vi "Define Cells names.vi"(8 "error in (no error)":errorcluster, 11 "Control-Client in":refnum<class "Control-Client.lvclass">) -> (0 "error out":errorcluster, 3 "Control-Client out":refnum<class "Control-Client.lvclass">)   [LabVIEW 2019, in "Control-Client.lvclass"]
uses:
  Control-Client.lvclass
  Control-Client.lvclass/Control-Client.ctl
panel:
  in  "Names of cells":string[](array[string])
  in  "stop":bool
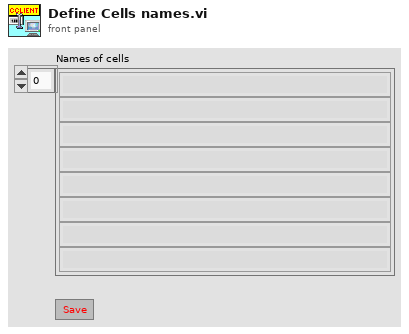
[diagram p1: front panel]
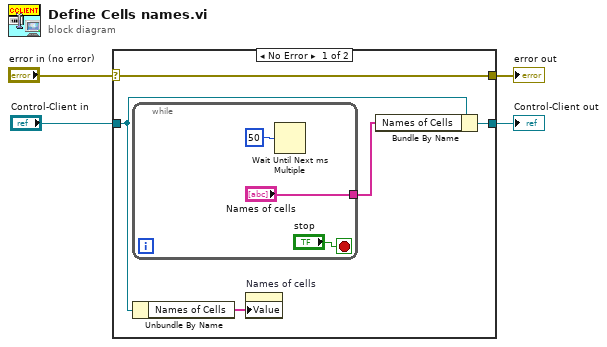
[diagram p0: block diagram]
diagram:
  n1 = case shown="No Error" "error in (no error)" {
    selector: "error in (no error)" -> [w9 w14]
    tunnel: [w9 w14] -> w3
    tunnel: [w5 w13] -> w1
    tunnel: "Control-Client in" -> [w8 w13]
    frame No Error {
      n2 = while {
        tunnel: ["Names of cells"] -> w6
        stop <- "stop" stop-if-true
        n3 = Wait Until Next ms Multiple(millisecond multiple=u32 50) -> ()  [unwired: 1 out]
      }
      n4 = Unbundle By Name(w8) -> ("Names of Cells"=w7:string[])
      n5 = property on="Names of cells" class="Arr (strict)"("Value"=w7) -> ()  [unwired: 2 in, 2 out]
      n6 = Bundle By Name(cluster=w8, "Names of Cells"=w6) -> (w5:refnum<class "Control-Client.lvclass">)
    }
    frame Error {
    }
  }
  "error out" <- w3
  "Control-Client out" <- w1
